vi "day 4 task 2.vi"() -> ()   [LabVIEW 2019]
panel:
  out "no. ranges that overlap at all":u64
  out "no. ranges that fully contain the other":u64
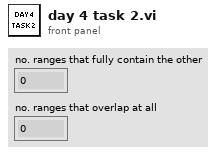
[diagram p1: front panel]
types:
  T1 = cluster{"first elf":cluster{"upper":i32, "lower":i32}, "second elf":cluster{"upper":i32, "lower":i32}}
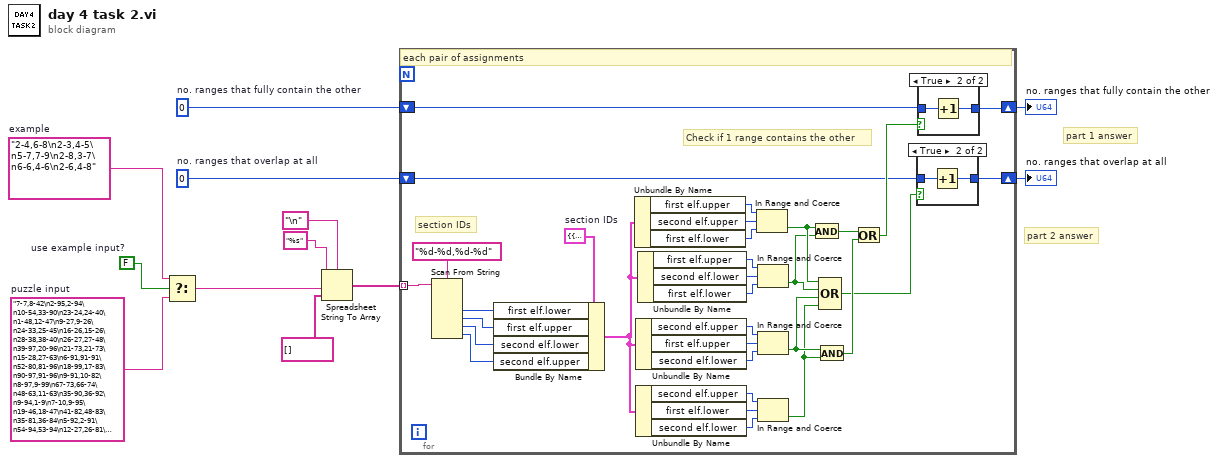
[diagram p0: block diagram]
diagram:
  w2 = u64 0  # no. ranges that overlap at all
  w4 = u64 0  # no. ranges that fully contain the other
  w7 = FALSE  # use example input?
  w8 = "7-7,8-42\n2-95,2-94\n10-54,33-90\n23-24,24-40\n1-48,12-47\n9-27,9-26\n24-33,25-45\n16-26,15-26\n28-38,38-40\n26-27,27-48\n39-97,20-96\n21-73,21-73\n15-28,27-63\n6-91,91-91\n52-80,81-96\n18-99,17-83\n90-97,91-96\n9-91,10-82\n8-97,9-99\n67-73,66-74\n48-63,11-63\n35-90,36-92\n9-94,1-9\n7-10,9-95\n19-46,18-47\n41-82,48-83\n35-81,36-84\n5-92,2-91\n54-94,53-94\n12-27,26-81\n17-26,8-14\n18-84,9-85\n49-64,65-82\n39-84,38-83\n20-65,64-66\n16-95,16-80\n31-36,37-78\n19-71,19-19\n12-90,11-89\n12-47,11-48\n10-11,10-74\n30-90,6-89\n17-26,16-25\n15-35,14-36\n29-29,28-28\n34-34,26-33\n11-26,12-76\n94-95,29-94\n62-65,62-64\n58-61,9-59\n12-75,11-13\n8-20,11-24\n66-95,66-86\n36-37,37-91\n6-17,16-18\n13-94,94-94\n83-96,75-92\n12-81,12-80\n4-68,3-46\n85-87,66-86\n8-31,30-37\n4-94,2-5\n14-30,33-84\n22-92,21-22\n4-95,20-95\n35-78,35-78\n8-80,8-8\n3-69,23-76\n11-98,10-96\n11-85,20-83\n24-58,11-31\n7-96,8-97\n66-77,78-97\n40-86,40-87\n53-79,53-79\n37-46,36-38\n1-91,1-92\n14-21,9-14\n15-37,38-38\n3-58,1-58\n59-85,51-86\n1-69,3-70\n3-74,36-75\n34-74,35-86\n8-98,7-75\n79-86,78-98\n23-97,23-93\n1-2,2-92\n68-77,68-78\n4-57,1-57\n99-99,53-96\n15-62,61-88\n13-65,9-14\n25-82,82-82\n48-54,47-77\n16-26,27-97\n16-18,17-91\n10-95,2-9\n98-99,7-98\n19-36,14-20\n6-30,7-84\n1-1,1-99\n24-52,11-51\n92-92,45-88\n88-89,88-90\n4-84,3-53\n37-52,36-38\n20-93,6-93\n63-63,17-62\n8-22,5-9\n52-77,52-52\n44-46,45-87\n14-82,13-74\n56-68,41-68\n80-80,16-80\n4-95,3-94\n57-95,63-96\n77-94,75-93\n55-91,91-91\n15-15,1-15\n44-98,45-45\n14-21,6-13\n4-42,2-4\n5-90,8-60\n32-62,33-50\n18-51,18-54\n4-30,3-4\n28-51,28-50\n93-96,31-94\n3-15,14-81\n15-74,84-89\n5-93,4-92\n1-5,6-90\n53-55,54-85\n20-90,20-57\n97-98,48-97\n27-48,26-36\n16-47,16-48\n94-96,88-94\n43-58,59-85\n88-90,10-84\n18-62,17-93\n14-97,14-98\n19-81,8-80\n13-94,12-89\n65-98,64-66\n36-48,35-49\n26-79,36-87\n54-62,53-69\n14-26,14-26\n18-71,70-71\n31-45,7-67\n3-94,1-4\n60-81,61-82\n16-66,66-66\n46-95,94-94\n10-89,10-90\n29-86,11-28\n55-96,54-56\n7-52,9-76\n65-93,83-92\n61-74,61-74\n72-93,93-93\n45-74,74-74\n19-98,20-98\n5-95,6-96\n21-96,96-97\n33-73,23-33\n68-85,15-42\n10-99,10-10\n4-96,93-97\n86-97,3-86\n46-86,47-87\n21-94,18-93\n64-64,28-64\n42-43,42-94\n52-97,53-98\n2-41,2-41\n12-80,11-13\n55-95,55-96\n12-35,21-36\n19-87,20-86\n56-67,37-57\n34-51,33-52\n9-92,8-91\n31-99,3-99\n23-24,24-84\n11-11,11-52\n12-72,11-46\n85-93,18-92\n33-90,99-99\n91-94,92-95\n14-68,68-69\n45-88,45-89\n7-89,4-6\n23-33,24-93\n35-84,46-83\n8-81,8-81\n50-72,40-71\n6-80,41-79\n8-64,5-7\n25-49,24-24\n43-96,7-42\n3-92,3-92\n6-46,1-45\n13-57,12-56\n55-62,32-63\n28-32,21-39\n5-6,5-46\n2-87,2-86\n10-83,8-82\n14-69,13-69\n67-69,68-89\n55-91,28-39\n23-30,29-58\n35-35,35-62\n48-63,49-65\n4-80,1-79\n2-60,2-61\n30-75,97-98\n15-95,14-40\n40-41,40-40\n69-96,27-96\n6-96,7-98\n14-98,13-15\n5-5,5-83\n2-92,3-91\n73-91,84-90\n3-97,90-96\n3-97,35-98\n73-93,73-74\n32-79,32-51\n44-80,44-79\n6-53,5-84\n41-48,42-49\n32-86,31-85\n4-86,4-86\n3-59,27-60\n24-93,10-23\n35-59,34-84\n8-93,9-9\n34-69,53-68\n64-91,63-64\n4-45,3-5\n81-88,43-87\n7-30,35-75\n47-78,5-46\n51-51,51-74\n20-67,49-76\n53-80,52-53\n2-37,1-98\n16-99,15-97\n97-97,6-97\n9-99,9-98\n38-93,24-55\n20-77,78-78\n10-76,75-76\n41-56,1-55\n39-93,39-91\n87-93,15-30\n9-98,9-85\n14-53,53-53\n70-94,11-95\n97-98,39-97\n50-81,71-72\n55-62,55-82\n9-21,9-9\n47-84,46-57\n1-32,3-31\n17-77,3-18\n20-69,20-68\n10-61,10-10\n18-97,97-98\n27-97,99-99\n10-60,1-60\n26-78,1-66\n4-10,11-11\n7-77,6-78\n29-75,74-75\n62-62,61-84\n3-82,82-82\n38-43,38-42\n2-84,3-85\n72-83,83-84\n40-92,98-98\n84-92,17-91\n36-85,14-35\n30-32,31-70\n11-61,12-12\n6-81,92-98\n16-93,16-93\n7-63,6-62\n4-98,4-97\n93-94,10-93\n19-30,18-30\n17-18,19-55\n53-98,50-98\n3-97,97-97\n2-97,2-98\n33-77,2-32\n52-53,10-52\n14-16,15-91\n29-99,17-98\n3-4,5-96\n4-92,3-4\n37-56,2-36\n28-52,26-99\n12-97,12-97\n14-43,44-72\n90-94,91-93\n5-80,10-81\n21-77,77-78\n39-91,42-90\n40-51,28-50\n4-91,5-78\n34-92,33-92\n6-8,5-99\n7-7,7-39\n54-88,53-53\n56-84,55-83\n7-80,6-8\n9-17,17-22\n19-50,51-53\n42-91,2-90\n26-27,27-69\n23-58,15-22\n22-92,25-93\n4-5,4-81\n75-89,76-76\n16-74,15-73\n3-70,4-69\n30-48,36-69\n23-40,23-94\n35-73,35-75\n78-86,31-87\n61-87,60-61\n72-91,2-92\n88-98,4-86\n14-25,13-17\n35-45,35-98\n7-92,7-99\n9-78,19-77\n16-92,12-42\n4-19,5-20\n1-95,3-96\n92-92,12-92\n80-80,80-84\n12-73,12-73\n4-92,5-93\n19-83,18-82\n12-13,12-14\n2-97,2-97\n6-93,7-58\n34-57,56-73\n6-39,13-98\n7-72,3-71\n11-86,13-86\n50-56,11-55\n12-31,19-19\n4-94,1-95\n44-93,1-94\n80-80,58-79\n7-95,7-96\n5-40,6-39\n7-57,19-57\n70-74,70-81\n7-91,1-91\n1-98,1-99\n1-98,56-61\n36-87,36-87\n1-43,8-44\n1-63,63-63\n2-91,1-82\n8-88,88-89\n53-54,2-53\n32-91,32-85\n3-88,88-89\n3-88,1-2\n33-71,29-34\n40-74,50-75\n8-12,11-53\n13-80,5-80\n2-12,4-11\n2-91,1-35\n4-77,3-76\n36-86,19-85\n27-53,28-52\n44-57,58-68\n61-89,58-88\n41-42,42-85\n91-92,27-91\n1-35,3-71\n40-40,10-40\n47-53,50-64\n77-78,31-77\n21-22,23-31\n19-69,18-70\n21-98,21-21\n24-70,24-70\n55-57,52-53\n53-84,53-53\n71-77,71-78\n13-48,7-47\n4-97,4-4\n4-28,37-73\n36-40,35-39\n9-18,28-90\n42-95,95-96\n11-21,7-20\n19-84,18-83\n5-69,1-4\n37-65,3-38\n2-98,1-99\n93-99,9-94\n44-93,44-93\n7-11,6-70\n8-94,93-95\n13-84,17-84\n11-73,30-74\n3-5,5-96\n55-80,79-91\n4-6,5-71\n74-77,74-78\n47-54,47-54\n52-72,73-80\n11-19,18-73\n42-44,43-83\n53-67,52-52\n2-42,18-86\n18-18,19-67\n12-91,12-95\n19-73,20-74\n47-97,96-98\n14-62,15-63\n14-69,3-70\n33-52,33-52\n32-63,62-64\n3-7,8-84\n47-48,12-47\n8-8,9-9\n43-92,20-20\n44-91,90-92\n62-68,63-71\n6-49,5-48\n14-24,3-23\n28-94,23-95\n82-91,27-82\n13-84,3-85\n1-92,1-87\n58-96,58-83\n99-99,7-98\n6-44,15-43\n72-72,17-71\n22-95,96-97\n10-92,10-92\n56-56,56-97\n79-81,80-83\n4-89,95-99\n10-76,14-72\n20-66,20-65\n4-76,4-77\n5-64,2-6\n17-78,4-77\n33-41,40-66\n46-54,46-72\n18-97,6-14\n1-99,21-96\n1-39,38-90\n15-25,7-17\n23-83,23-82\n23-82,24-60\n8-54,54-83\n42-60,12-31\n25-96,13-87\n15-20,14-98\n80-80,21-79\n2-88,2-2\n91-94,32-90\n12-98,10-12\n9-83,10-84\n17-39,19-40\n39-48,40-74\n20-84,1-19\n42-77,42-76\n29-33,31-34\n11-86,12-88\n2-99,2-99\n38-95,19-54\n4-4,5-90\n3-93,21-93\n58-88,88-89\n15-98,9-12\n9-76,9-75\n9-9,10-32\n1-30,1-31\n2-81,2-82\n28-72,89-97\n4-40,39-90\n23-54,53-55\n26-95,27-95\n4-84,8-83\n24-26,28-31\n32-57,32-72\n46-61,36-60\n22-80,21-21\n9-73,8-74\n15-30,21-64\n42-97,42-42\n20-31,20-20\n5-9,9-97\n39-83,11-84\n45-83,44-84\n72-95,71-73\n12-90,8-13\n5-7,7-89\n79-81,80-81\n19-20,20-58\n4-30,3-5\n30-67,66-68\n2-2,5-96\n23-97,23-93\n45-98,43-97\n53-93,53-92\n10-74,9-10\n66-70,24-66\n15-53,48-65\n31-96,31-96\n11-79,10-80\n43-76,43-53\n74-93,7-94\n7-45,8-79\n76-85,85-85\n1-56,56-56\n85-90,86-90\n24-43,12-43\n8-9,8-53\n56-94,55-57\n28-76,29-77\n12-90,10-13\n38-90,40-42\n48-99,59-98\n81-81,18-81\n73-73,72-87\n29-94,94-95\n7-46,46-46\n94-94,3-94\n4-89,4-89\n66-71,67-70\n19-62,63-87\n16-16,16-34\n22-98,8-97\n43-87,42-44\n5-35,1-34\n32-56,95-97\n7-46,6-98\n76-88,67-75\n7-62,6-8\n29-75,30-76\n55-99,34-55\n18-57,3-30\n91-92,8-91\n4-95,98-98\n55-55,45-57\n35-88,34-87\n21-98,21-99\n42-44,43-76\n14-15,14-76\n36-90,36-87\n8-14,7-14\n26-99,25-98\n28-50,14-39\n39-64,39-95\n3-50,2-22\n58-84,57-59\n10-50,9-11\n14-42,13-15\n51-65,50-54\n47-82,83-93\n76-76,12-76\n14-38,3-37\n15-44,14-45\n32-97,4-98\n30-61,31-62\n42-84,5-37\n20-99,19-21\n13-37,14-45\n19-72,11-20\n22-98,22-98\n61-96,35-62\n54-70,46-69\n70-82,68-74\n25-73,25-73\n42-44,41-46\n27-97,26-27\n1-80,1-81\n6-98,3-5\n60-61,37-60\n20-80,5-21\n29-78,30-44\n8-76,7-75\n45-62,45-96\n8-99,7-7\n46-72,46-46\n68-86,67-83\n9-25,8-24\n11-55,10-12\n19-82,20-83\n20-98,19-97\n57-59,55-59\n80-82,81-87\n5-85,84-86\n80-94,2-63\n29-81,80-82\n35-35,36-71\n41-45,40-77\n38-97,11-98\n2-99,98-99\n24-26,25-48\n60-61,35-60\n45-70,44-84\n17-49,49-50\n69-99,68-98\n25-70,70-99\n47-50,39-51\n67-85,67-85\n47-98,47-99\n98-98,56-98\n21-98,3-99\n5-94,1-2\n51-98,19-97\n52-72,73-77\n36-74,24-44\n8-18,70-95\n7-83,96-96\n1-94,2-95\n10-24,25-44\n14-53,13-43\n41-73,63-66\n56-59,57-61\n65-66,64-77\n42-42,41-88\n3-6,2-4\n52-93,51-92\n22-84,21-85\n20-99,8-20\n6-84,84-85\n53-66,30-66\n27-31,13-29\n12-55,11-12\n7-85,76-86\n94-99,53-93\n2-3,4-85\n35-37,36-41\n13-78,89-93\n22-84,21-83\n93-95,11-68\n15-72,53-94\n5-58,5-5\n98-98,55-92\n20-59,21-60\n6-96,8-96\n7-33,7-32\n69-69,36-68\n24-97,10-96\n56-96,63-95\n3-61,3-94\n35-59,34-39\n21-52,21-53\n26-92,26-27\n53-81,52-82\n17-63,16-18\n42-42,42-56\n7-67,7-8\n43-92,43-92\n2-51,25-57\n5-7,6-90\n14-71,71-85\n16-87,2-8\n24-51,18-44\n49-51,50-60\n3-98,1-4\n3-96,1-2\n8-76,8-95\n32-95,32-94\n46-87,19-86\n77-96,28-66\n10-71,71-94\n3-97,3-96\n10-61,1-11\n13-81,14-82\n26-99,27-69\n40-69,40-69\n9-61,1-8\n19-23,22-99\n3-6,6-85\n24-95,94-96\n76-77,34-77\n6-79,6-7\n22-68,21-60\n12-84,84-85\n7-72,7-81\n10-74,49-73\n47-89,46-48\n2-2,2-96\n20-82,36-81\n25-62,24-61\n14-25,24-88\n10-57,28-57\n58-89,59-93\n5-9,9-10\n18-18,18-90\n62-84,24-85\n8-62,8-63\n55-90,8-55\n2-93,1-92\n35-60,59-75\n24-93,32-92\n35-69,7-70\n4-93,5-92\n27-45,18-27\n30-98,24-24\n7-90,6-91\n72-93,72-83\n8-98,6-95\n35-75,35-74\n3-58,2-33\n17-98,98-98\n5-90,3-70\n13-25,12-14\n17-61,18-62\n25-54,12-53\n5-79,78-80\n8-85,87-94\n1-2,1-96\n55-64,55-65\n51-60,59-89\n2-54,2-2\n12-96,12-92\n18-99,17-62\n50-93,45-92\n41-91,41-91\n8-86,9-75\n34-46,47-47\n89-90,30-90\n65-88,65-88\n75-75,8-75\n1-93,6-93\n7-7,6-86\n94-98,37-92\n8-72,72-72\n14-33,14-14\n30-52,53-82\n25-81,17-25\n10-70,44-85\n9-34,34-45\n31-94,30-92\n55-84,55-83\n3-86,4-89\n27-32,28-32\n21-50,51-60\n9-80,27-81\n17-72,17-70\n49-49,51-87\n32-42,35-41\n3-6,4-40\n11-13,12-90\n42-63,18-64\n50-91,12-92\n7-90,90-98\n43-99,10-98\n53-63,55-57\n62-83,84-84\n1-58,4-82\n36-62,36-71\n80-91,8-77\n37-46,5-47\n5-7,6-78\n25-60,24-24\n16-62,16-95\n10-11,10-23\n2-13,12-53\n96-96,41-95\n33-48,32-48\n29-79,29-67\n17-30,31-90\n3-96,1-97\n2-99,6-98\n58-98,45-59\n72-74,72-72\n50-94,49-93\n2-6,13-87\n47-92,98-99\n49-90,33-91\n65-67,54-66\n8-40,2-7\n41-47,41-41\n12-87,11-43\n3-81,2-82\n13-25,13-25\n21-66,55-65\n3-50,34-51\n42-93,28-43\n57-89,57-57\n25-95,99-99\n7-98,97-98\n61-62,44-61\n70-71,3-70\n6-71,21-70\n16-54,8-17\n33-78,53-70\n19-21,20-70\n25-88,26-99\n2-35,34-71\n84-96,23-77\n6-97,4-31\n21-87,25-47\n31-38,38-82\n4-91,4-92\n81-81,1-81\n6-94,94-95\n2-11,1-3\n6-98,4-98\n41-74,74-74\n30-96,97-97\n15-91,15-92\n32-97,31-94\n9-48,6-47\n4-75,4-74\n33-49,49-49\n58-95,39-94\n6-99,5-53\n69-72,70-73\n2-91,89-90\n8-8,8-21\n2-11,9-10\n5-67,5-5\n21-58,20-59\n3-97,1-3\n56-62,57-76\n26-93,92-94\n98-98,95-96\n59-96,60-80\n76-94,51-77\n76-99,76-98\n10-83,28-84\n1-91,91-91\n9-58,3-57\n54-70,55-69\n70-71,8-71\n6-9,9-96\n53-65,53-66\n9-84,11-85\n29-77,29-78\n17-65,16-80\n16-74,2-73\n46-91,77-92\n11-66,12-25\n4-81,80-82\n5-48,52-56\n8-94,6-11\n13-88,89-99\n97-99,3-98\n83-85,72-86\n3-4,4-10\n21-43,21-89\n14-28,15-39\n79-79,7-79\n20-20,21-95\n4-80,8-95\n61-92,62-95\n37-37,11-36\n19-81,20-88\n20-40,20-40\n55-97,54-98\n72-93,10-94\n13-94,14-98\n15-16,16-30\n43-62,58-63\n1-2,3-90\n3-77,3-77\n5-39,2-38\n49-74,82-87\n17-24,23-24\n82-84,12-83\n11-90,31-90\n41-41,42-95\n53-73,79-92\n10-92,11-91\n64-69,64-64\n90-97,28-76\n8-98,8-95\n10-84,10-11\n27-78,20-79\n59-59,58-99\n15-54,24-90\n18-36,9-28\n51-52,24-53\n90-93,47-78\n8-17,16-77\n3-76,83-98\n25-62,24-25\n10-13,14-17\n5-35,10-34\n11-98,10-98\n22-70,22-71\n5-96,1-98\n13-63,30-62\n13-42,47-92\n2-98,2-89\n3-7,6-97\n42-47,42-42\n5-63,62-64\n13-96,15-97\n88-88,33-88\n49-70,48-69\n9-96,95-97\n3-86,45-74\n12-67,12-12\n7-87,8-92\n48-97,17-67\n40-60,38-59\n4-10,13-15\n8-81,9-80\n1-73,1-26\n1-3,3-74\n54-54,55-55\n24-34,35-93\n44-65,43-66\n15-15,15-98\n11-85,53-87\n13-73,13-28\n1-5,7-49\n8-54,8-89\n4-38,3-37\n43-94,93-95\n9-96,8-10\n40-77,27-41\n38-40,39-69\n4-62,52-67\n35-47,17-46\n33-92,30-32\n32-90,90-90\n2-87,2-87\n8-8,8-90\n65-69,69-70\n86-86,1-86\n71-93,4-51\n41-71,57-71\n68-85,60-84\n3-97,7-97\n98-98,12-98\n23-71,22-65\n42-54,44-54\n77-98,24-97\n81-84,83-84\n5-93,5-92\n1-99,97-98\n25-98,17-26\n19-99,19-97\n11-93,11-93\n12-95,10-13\n34-39,34-57\n25-39,14-38\n11-48,11-48\n84-91,1-83\n22-95,21-21\n1-1,3-91\n57-95,95-95\n12-99,6-98\n12-71,12-23\n89-96,13-70\n64-74,1-75\n19-91,19-90\n93-94,4-93\n20-89,89-89\n90-92,1-91\n7-98,8-28\n1-47,2-48\n99-99,1-99\n32-74,32-74\n5-8,4-89\n5-94,2-95\n58-92,91-92\n35-49,48-49\n24-73,74-92\n90-91,4-91\n24-90,18-91\n62-70,63-69\n16-88,87-88\n6-8,7-93\n7-98,8-67\n12-86,11-86\n64-86,63-63\n48-73,29-76\n3-35,31-34\n59-68,59-69\n11-98,10-12\n17-17,17-87\n6-88,6-87\n6-63,80-92"  # puzzle input
  w9 = "2-4,6-8\n2-3,4-5\n5-7,7-9\n2-8,3-7\n6-6,4-6\n2-6,4-8"  # example
  # "part 2 answer"
  # "part 1 answer"
  n1 = Select(t=w9, s=w7, f=w8) -> (s? t:f=w6:string)
  n2 = Spreadsheet String To Array(delimiter (Tab)="\n", format string="%s", spreadsheet string=w6, array type (2D Dbl)=string[] []) -> (array=w5:string[])
  n3 = for {
    tunnel: w5 -> [w44] mode=indexing
    shift-right: [w39] -> w3
    shift-left: w4 -> [w40]
    shift-right: [w14] -> w1
    shift-left: w2 -> [w15]
    w37 = T1 {"first elf"={"upper"=0, "lower"=0}, "second elf"={"upper"=0, "lower"=0}}  # section IDs
    # "section IDs"
    # "Check if 1 range contains the other"
    # "each pair of assignments"
    n4 = Scan From String(format string="%d-%d,%d-%d", input string=w44) -> (output 1=w36:i32, output 2=w35:i32, output 3=w34:i32, output 4=w33:i32)  [unwired: 6 in, 3 out]
    n5 = Bundle By Name(cluster=w37, "first elf.lower"=w36, "first elf.upper"=w35, "second elf.lower"=w34, "second elf.upper"=w33) -> (w23:T1)
    n6 = Unbundle By Name(w23) -> ("first elf.upper"=w30:i32, "second elf.upper"=w29:i32, "first elf.lower"=w32:i32)
    n7 = Unbundle By Name(w23) -> ("second elf.upper"=w26:i32, "first elf.upper"=w25:i32, "second elf.lower"=w24:i32)
    n8 = Unbundle By Name(w23) -> ("second elf.upper"=w22:i32, "first elf.lower"=w20:i32, "second elf.lower"=w21:i32)
    n9 = Unbundle By Name(w23) -> ("first elf.upper"=w31:i32, "second elf.lower"=w27:i32, "first elf.lower"=w28:i32)
    n10 = In Range and Coerce(upper limit=w30, x=w29, lower limit=w32) -> (In Range?=w19:bool)  [unwired: 1 out]
    n11 = In Range and Coerce(upper limit=w31, x=w27, lower limit=w28) -> (In Range?=w18:bool)  [unwired: 1 out]
    n12 = In Range and Coerce(upper limit=w26, x=w25, lower limit=w24) -> (In Range?=w17:bool)  [unwired: 1 out]
    n13 = In Range and Coerce(upper limit=w22, x=w20, lower limit=w21) -> (In Range?=w16:bool)  [unwired: 1 out]
    n14 = And(x=w19, y=w18) -> (x .and. y?=w42:bool)
    n15 = And(x=w17, y=w16) -> (x .and. y?=w41:bool)
    n16 = Compound Arithmetic op=OR(w19, w18, w17, w16) -> (w13:bool)
    n17 = Or(x=w42, y=w41) -> (x .or. y?=w38:bool)
    n18 = case shown="True" w13 {
      tunnel: w15 -> [w45 w47]
      tunnel: [w45 w46] -> w14
      frame False {
      }
      frame True {
        n19 = Increment(x=w47) -> (x+1=w46:u64)
      }
    }
    n20 = case shown="True" w38 {
      tunnel: w40 -> [w48 w50]
      tunnel: [w48 w49] -> w39
      frame False {
      }
      frame True {
        n21 = Increment(x=w50) -> (x+1=w49:u64)
      }
    }
  }
  "no. ranges that fully contain the other" <- w3
  "no. ranges that overlap at all" <- w1
